vi "anCLASS.vi"(7 "Set? (f)":bool, 11 "MyPlugins.lvlib In":refnum<class "MyPluginsBase.lvclass">) -> (3 "MyPlugins.lvlib Out":refnum<class "MyPluginsBase.lvclass">)   [LabVIEW 2014, in "MyPluggableModule.lvlib"]
uses:
  MyPlugins/MyPluginBaseClass/MyPluginsBase.lvclass
  MyPluggableModule.lvlib
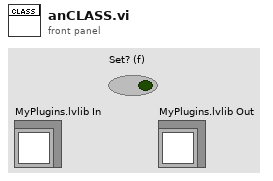
[diagram p1: front panel]
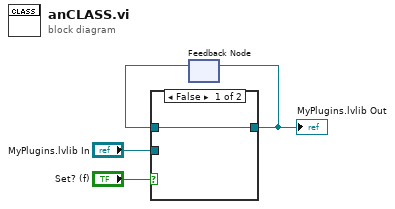
[diagram p0: block diagram]
diagram:
  n1 = feedback #1() -> (w1:refnum<class "MyPluginsBase.lvclass">)  [unwired: 1 in]
  n2 = case shown="False" "Set? (f)" {
    tunnel: "MyPlugins.lvlib In" -> [_ w6]
    tunnel: [w5 w6] -> w2
    tunnel: w1 -> [w5 _]
    frame False {
    }
    frame True {
    }
  }
  "MyPlugins.lvlib Out" <- w2
  n3 = feedback-in #1(w2) -> ()
